vi "Window Memory write from DMA - Host.vi"(8 "error in":errorcluster, 10 "Enum":T1(ring)=enum."Hamming", 11 "FPGA VI Reference In":refnum<k20>) -> (0 "FPGA VI Reference Out":refnum<k20>, 2 "Window Array":fxp<+,8,1>[](array[numeric]), 3 "error out":errorcluster, 6 "Write memory complete":bool)   [LabVIEW 2014]
uses:
  <vilib>/rvi/interface/common/niFpgaWaitOnOcc.vi
  <vilib>/Utility/error.llb/Error Cluster From Error Code.vi
  <vilib>/rvi/errors/niLvFpgaAdjustHostInterfaceError.vi
  <vilib>/RVI Host/nirviSupport.llb/nirviErrorClusterFromErrorCode.vi
  <vilib>/rvi/interface/nirviMethod/nirviMethod.xnode
  <vilib>/rvi/errors/niLvFpgaMergeErrorWithErrorCode.vi
  <vilib>/rvi/interface/nirviMethod/StockFPGA_InlinedMethodWaitForSingleIRQ.vi
  <vilib>/FPGAPlugInAG/Dynamic/niLvFpga_WaitOnIrq_Dynamic.vi
  <vilib>/FPGAPlugInAG/Dynamic/niLvFpga_AcknowledgeIrq_Dynamic.vi
  <vilib>/FPGAPlugInAG/Dynamic/niLvFpga_ConfigureFifo_Dynamic.vi
  <vilib>/FPGAPlugInAG/Dynamic/niLvFpga_StartFifo_Dynamic.vi
  <vilib>/FPGAPlugInAG/Dynamic/niLvFpga_WriteFifo_Dynamic.vi
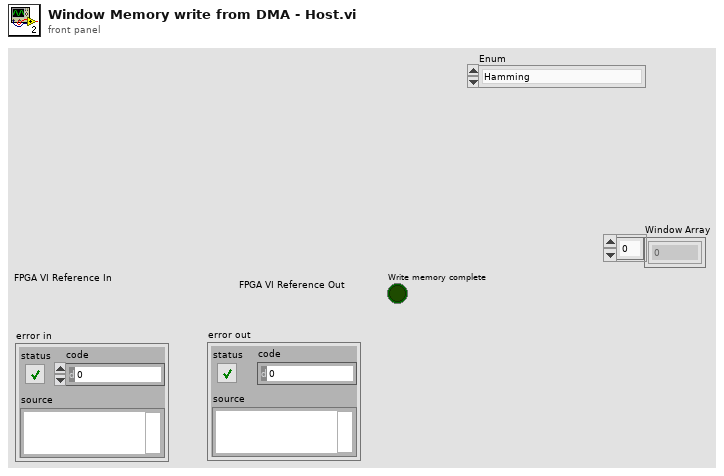
[diagram p1: front panel]
types:
  T1 = enum16{"None", "Hanning", "Hamming", "Blackman", "Blackman-Harris"}
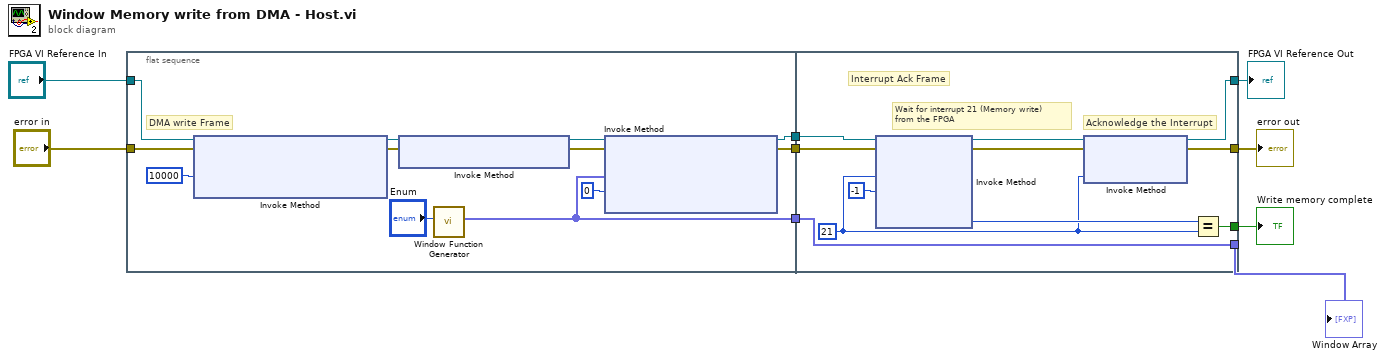
[diagram p0: block diagram]
diagram:
  n1 = flat-sequence {
    tunnel: [w15] -> w9
    tunnel: [w14] -> w8
    tunnel: "error in" -> [w13]
    tunnel: "FPGA VI Reference In" -> [w12]
    tunnel: [w11] -> w7
    tunnel: [w26] -> w2
    tunnel: [w27] -> w6
    tunnel: w9 -> [w31]
    tunnel: w8 -> [w32]
    tunnel: [w23] -> w5
    tunnel: [w22] -> w1
    tunnel: w7 -> [w22]
    frame #0 {
      # "DMA write Frame"
      n2 = xnode "Invoke Method"("FPGA VI Reference In"=w12, "error in"=w13, "Requested Depth"=u32 10000) -> ("FPGA VI Reference Out"=w20:refnum<k20>, "error out"=w19:errorcluster)  [unwired: 1 out]
      n3 = xnode "Invoke Method"("FPGA VI Reference In"=w20, "error in"=w19) -> ("FPGA VI Reference Out"=w17:refnum<k20>, "error out"=w18:errorcluster)
      n4 = call "Window Function Generator.vi"("Enum"="Enum") -> ("Window Array"=w11:fxp<+,8,1>[])  [unwired: 10 in]
      n5 = xnode "Invoke Method"("FPGA VI Reference In"=w17, "error in"=w18, "Data"=w11, "Timeout (ms)"=0) -> ("FPGA VI Reference Out"=w15:refnum<k20>, "error out"=w14:errorcluster)  [unwired: 1 out]
    }
    frame #1 {
      w24 = 21 ("IRQ Number(s)")
      # "Acknowledge the Interrupt"
      # "Wait for interrupt 21 (Memory write)\nfrom the FPGA"
      # "Interrupt Ack Frame"
      n6 = xnode "Invoke Method"("FPGA VI Reference In"=w31, "error in"=w32, "IRQ Number(s)"=w24, "Timeout (ms)"=-1) -> ("FPGA VI Reference Out"=w28:refnum<k20>, "error out"=w29:errorcluster, "IRQ(s) Asserted"=w25:i32)  [unwired: 1 out]
      n7 = xnode "Invoke Method"("FPGA VI Reference In"=w28, "error in"=w29, "IRQ Number(s)"=w24) -> ("FPGA VI Reference Out"=w26:refnum<k20>, "error out"=w27:errorcluster)
      n8 = Equal?(x=w25, y=w24) -> (x = y?=w23:bool)
    }
  }
  "error out" <- w6
  "Write memory complete" <- w5
  "FPGA VI Reference Out" <- w2
  "Window Array" <- w1
